vi "SincronizacionMain.vi"(7 "max":i64, 8 "error in":errorcluster, 9 "existe archivo":bool, 11 "semaphore":T1) -> (0 "error out":errorcluster, 1 "JSON":string, 2 "HTTP Response Code":i32, 3 "semaphore out":T1)   [LabVIEW 2015]
uses:
  <vilib>/addons/JSON API/JSON Array/Set JSON Array.vi
  <vilib>/addons/JSON API/JSON Value/Get as JSON string.vi
panel:
  out "size(s)":i32
  out "Boolean":bool
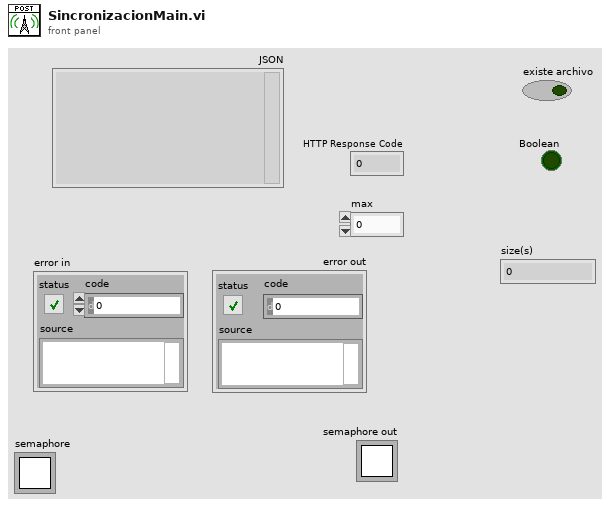
[diagram p1: front panel]
types:
  T1 = typedef "Semaphore RefNum" = refnum<k1>
  T2 = cluster{"tdms control out":refnum<k34>, "tdms historial out":refnum<k34>, "tdms sinc out":refnum<k34>}
  T3 = cluster{u32, dbl, dbl, dbl, dbl, dbl, dbl, dbl, dbl, dbl, dbl, dbl}[]
  T4 = cluster{u32, dbl, dbl, dbl, dbl, dbl, dbl, dbl, dbl, dbl, dbl, dbl, dbl, dbl, dbl, dbl, dbl, dbl, dbl, dbl}[]
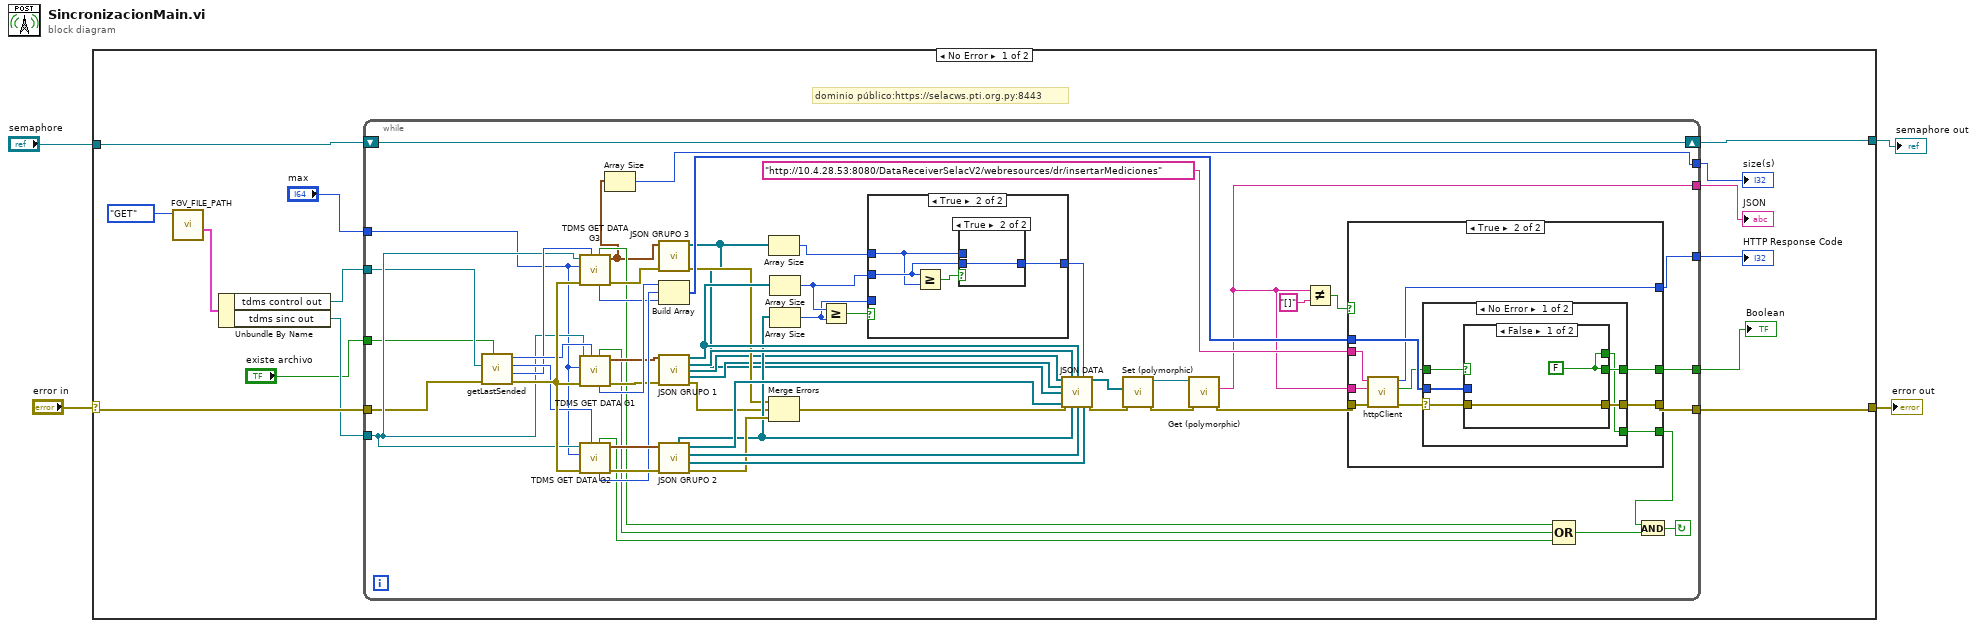
[diagram p0: block diagram]
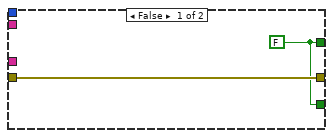
[diagram p2: hidden frame]
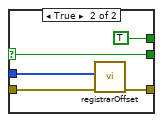
[diagram p3: hidden frame]
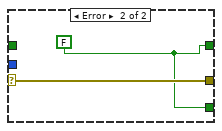
[diagram p4: hidden frame]
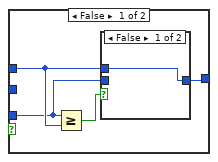
[diagram p5: hidden frame]
diagram:
  n1 = case shown="No Error" "error in" {
    selector: "error in" -> [w18 w116]
    tunnel: [w17 w116] -> w3
    tunnel: "semaphore" -> [w12 w115]
    tunnel: [w11 w115] -> w1
    frame No Error {
      # "dominio público:https://selacws.pti.org.py:8443"
      n2 = call "FGV_FILE_PATH.vi"("Function"=enum16{"GET", "SET"}."GET") -> ("Data Out"=w13:T2)  [unwired: 10 in]
      n3 = Unbundle By Name(w13) -> ("tdms control out"=w15:refnum<k34>, "tdms sinc out"=w14:refnum<k34>)
      n4 = while {
        tunnel: w15 -> [w48]
        tunnel: w14 -> [w49]
        tunnel: w18 -> [w47]
        tunnel: [w46] -> w17
        tunnel: "max" -> [w28]
        tunnel: "existe archivo" -> [w27]
        shift-right: [w50] -> w11
        shift-left: w12 -> [w50]
        tunnel: [w26] -> w8
        tunnel: [w25] -> w7
        tunnel: [w24] -> w6
        tunnel: [w23] -> w5
        stop <- w22 continue-if-true
        n5 = call "getLastSended.vi"("existe archivo"=w27, "error in"=w47, "tdms file"=w48) -> ("error out"=w60:errorcluster, "grupo 3"=w54:i32, "grupo 2"=w55:i32, "grupo 1"=w56:i32)  [unwired: 5 in]
        n6 = call "TDMS GET DATA G3.vi"("OffSet In"=w54, "error in"=w60, "max"=w28, "tdms file In"=w49) -> ("error out 2"=w73:errorcluster, "Result"=w20:T3, "lengh"=w51:i64, "Repetir"=w37:bool)  [unwired: 4 in]
        n7 = call "TDMS GET DATA G1.vi"("OffSet In"=w56, "error in"=w60, "max"=w28, "tdms file In"=w49) -> ("error out"=w42:errorcluster, "Result"=w43:cluster{u32, dbl, dbl, dbl, dbl}[], "lengh"=w52:i64, "Repetir"=w38:bool)  [unwired: 4 in]
        n8 = call "TDMS GET DATA G2.vi"("OffSet In"=w55, "error in"=w60, "max"=w28, "tdms file In"=w49) -> ("error out"=w74:errorcluster, "Grupo 2"=w75:T4, "lengh"=w53:i64, "Repetir"=w39:bool)  [unwired: 4 in]
        n9 = Array Size(array=w20) -> (size(s)=w24:i32)
        n10 = call "JSON GRUPO 3.vi"("error in"=w73, "Result"=w20) -> ("error IO"=w33:errorcluster, "Generador"=w19:refnum<class "JSON Object.lvclass">[])  [unwired: 8 in]
        n11 = Build Array(w52, w53, w51) -> (w59:i64[])
        n12 = call "JSON GRUPO 1.vi"("Result"=w43, "error in"=w42) -> ("PAR"=w41:refnum<class "JSON Object.lvclass">[], "Humedad R."=w40:refnum<class "JSON Object.lvclass">[], "Temp Amb"=w32:refnum<class "JSON Object.lvclass">[], "Temp Panel"=w31:refnum<class "JSON Object.lvclass">[], "error out"=w30:errorcluster)  [unwired: 9 in]
        n13 = call "JSON GRUPO 2.vi"("error in"=w74, "Grupo in"=w75) -> ("error out"=w58:errorcluster, "alarmas"=w70:refnum<class "JSON Array.lvclass">[], "JSON BAT"=w71:refnum<class "JSON Object.lvclass">[], "JSON CARGA"=w72:refnum<class "JSON Array.lvclass">[], "JSON FV"=w34:refnum<class "JSON Object.lvclass">[])  [unwired: 5 in]
        n14 = Array Size(array=w19) -> (size(s)=w36:i32)
        n15 = Merge Errors(w33, w30, w58) -> (w57:errorcluster)
        n16 = Array Size(array=w41) -> (size(s)=w69:i32)
        n17 = Array Size(array=w34) -> (size(s)=w68:i32)
        n18 = Greater Or Equal?(x=w69, y=w68) -> (x >= y?=w35:bool)
        n19 = case shown="True" w35 {
          tunnel: w69 -> [_ w111]
          tunnel: w68 -> [w103 _]
          tunnel: w36 -> [w104 w109]
          tunnel: [w105 w110] -> w67
          frame False {
            n20 = Greater Or Equal?(x=w103, y=w104) -> (x >= y?=w106:bool)
            n21 = case shown="False" w106 {
              tunnel: [w107 w108] -> w105
              tunnel: w104 -> [w107 _]
              tunnel: w103 -> [_ w108]
              frame False {
              }
              frame True {
              }
            }
          }
          frame True {
            n22 = Greater Or Equal?(x=w111, y=w109) -> (x >= y?=w112:bool)
            n23 = case shown="True" w112 {
              tunnel: w111 -> [_ w114]
              tunnel: [w113 w114] -> w110
              tunnel: w109 -> [w113 _]
              frame False {
              }
              frame True {
              }
            }
          }
        }
        n24 = call "JSON DATA.vi"("Temp Amb"=w32, "Humedad R."=w40, "PAR"=w41, "Numeric"=w67, "Temp Panel"=w31, "Generador"=w19, "JSON CARGA"=w72, "error in"=w57, "JSON FV"=w34, "JSON BAT"=w71, "alarmas"=w70) -> ("Array"=w66:refnum<class "JSON Object.lvclass">[], "error out"=w64:errorcluster)  [unwired: 3 in]
        n25 = call-poly <vilib>:"Set (polymorphic).vi"("error in (no error)"=w64, "Array"=w66) -> ("error out"=w63:errorcluster, "JSON Array out"=w65:refnum<class "JSON Array.lvclass">)  [unwired: 8 in]
        n26 = call-poly <vilib>:"Get (polymorphic).vi"("error in (no error)"=w63, "JSON Value in"=w65) -> ("error out"=w62:errorcluster, "String"=w26:string)  [unwired: 8 in]
        n27 = Not Equal?(x=w26, y="[]") -> (x != y?=w44:bool)
        n28 = case shown="True" w44 {
          tunnel: w62 -> [w77 w87]
          tunnel: "http://10.4.28.53:8080/DataReceiverSelacV2/webresources/dr/insertarMediciones" ("URI") -> [_ w86]
          tunnel: w59 -> [_ w85]
          tunnel: [w77 w82] -> w46
          tunnel: w26 -> [_ w81]
          tunnel: [_ w80] -> w25
          tunnel: [w76 w79] -> w23
          tunnel: [w76 w78] -> w21
          frame False {
            w76 = FALSE
          }
          frame True {
            n29 = call "httpClient.vi"("error in"=w87, "data"=w81, "URI"=w86) -> ("error out"=w84:errorcluster, "code create"=w83:bool, "HTTP Response Code"=w80:i32)  [unwired: 6 in]
            n30 = case shown="No Error" w84 {
              selector: w84 -> [w90 w102]
              tunnel: w85 -> [w93 _]
              tunnel: [w92 w102] -> w82
              tunnel: w83 -> [w91 _]
              tunnel: [w88 w101] -> w78
              tunnel: [w89 w101] -> w79
              frame No Error {
                n31 = case shown="False" w91 {
                  selector: w91 -> [_ w97]
                  tunnel: w93 -> [_ w98]
                  tunnel: [w95 w100] -> w92
                  tunnel: w90 -> [w95 w99]
                  tunnel: [w94 w97] -> w89
                  tunnel: [w94 TRUE] -> w88
                  frame False {
                    w94 = FALSE
                  }
                  frame True {
                    n32 = call "registrarOffset.vi"("error in (no error)"=w99, "Offsets"=w98) -> ("error out"=w100:errorcluster)  [unwired: 8 in, 1 out]
                  }
                }
              }
              frame Error {
                w101 = FALSE
              }
            }
          }
        }
        n33 = Compound Arithmetic op=OR(w37, w38, w39) -> (w29:bool)
        n34 = And(x=w21, y=w29) -> (x .and. y?=w22:bool)
      }
      "JSON" <- w8
      "HTTP Response Code" <- w7
      "size(s)" <- w6
      "Boolean" <- w5
    }
    frame Error {
    }
  }
  "error out" <- w3
  "semaphore out" <- w1
